vi "Screw Launcher.vi"(9 "Sub Panel":refnum<vi>, 10 "Screw ID":string="Secondary", 11 "Feeder Actor In":refnum<class "Feeder.lvclass">) -> (2 "Nested Actor's Enqueuer":refnum<class "Message Enqueuer.lvclass">, 3 "Feeder Actor Out":refnum<class "Feeder.lvclass">)   [LabVIEW 2018, in "Feeder Actor.lvlib" / "Screw.lvclass"]
uses:
  Screw.lvclass
  <vilib>/ActorFramework/Message Enqueuer/Message Enqueuer.lvclass
  Feeder/Feeder.lvclass
  C:/Program Files/National Instruments/LabVIEW 2018/vi.lib/MGI/Panel Manager/Panel Actor/Panel Actor/Panel Actor.lvclass
  Screw.lvclass/Screw.ctl
  <vilib>/MGI/Panel Manager/Panel/Panel/Subpanel/Subpanel.lvclass
  C:/Program Files/National Instruments/LabVIEW 2018/vi.lib/MGI/Panel Manager/Panel/Panel/Panel.lvclass
  <vilib>/DAQmx/create/channels.llb/DAQmx Create Channel (CO-Pulse Generation-Frequency).vi
  <vilib>/MGI/Panel Manager/Panel/Panel/Subpanel/Subpanel.vi
  <vilib>/DAQmx/configure/timing.llb/DAQmx Timing (Implicit).vi
  <vilib>/MGI/Panel Manager/Panel/Panel.lvlib
  <vilib>/MGI/Panel Manager/Panel Actor/Panel Actor/Panel Actor.lvclass
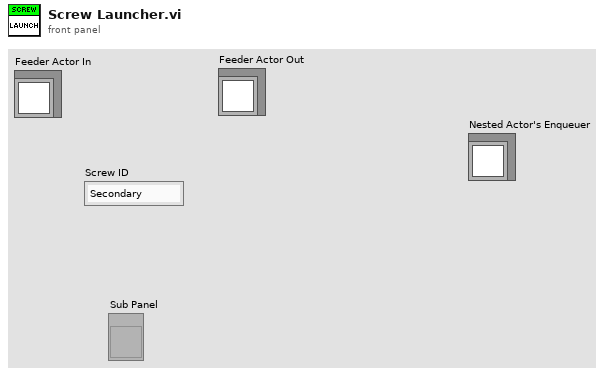
[diagram p1: front panel]
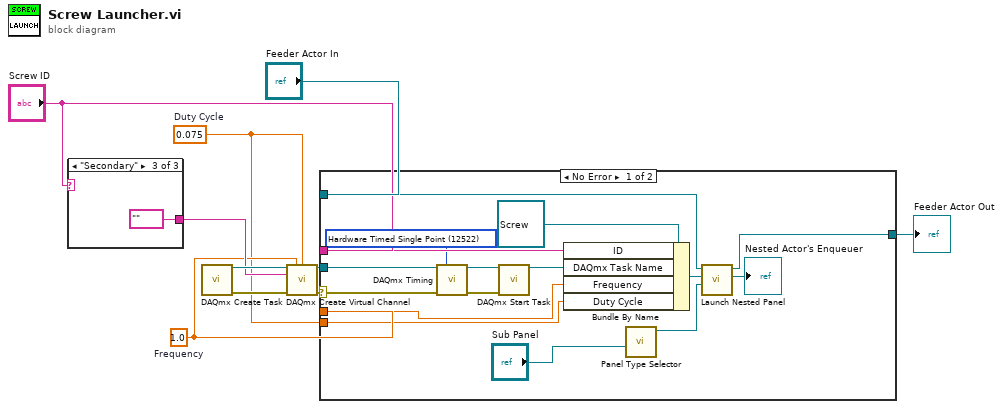
[diagram p0: block diagram]
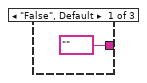
[diagram p2: hidden frame]
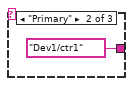
[diagram p3: hidden frame]
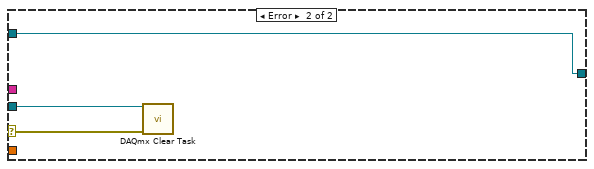
[diagram p4: hidden frame]
diagram:
  w1 = 0.075  # Duty Cycle
  w2 = 1.0  # Frequency
  n1 = case shown="\"Secondary\"" "Screw ID" {
    tunnel: [tag "" ("Counter(s) 2") tag "Dev1/ctr1" ("Counter(s) 2") tag "" ("Counter(s) 2")] -> w5
    frame "False", Default {
    }
    frame "Primary" {
    }
    frame "Secondary" {
    }
  }
  n2 = call <vilib>:"DAQmx Create Task.vi"() -> ("task out"=w7:refnum<k21>, "error out"=w6:errorcluster)  [unwired: 14 in]
  n3 = call-poly <vilib>:"DAQmx Create Virtual Channel.vi"("task in"=w7, "frequency"=w2, "duty cycle"=w1, "counter"=w5, "error in"=w6) -> ("task out"=w3:refnum<k21>, "error out"=w4:errorcluster)  [unwired: 9 in]
  n4 = case shown="No Error" w4 {
    selector: w4 -> [w19 w30]
    tunnel: "Screw ID" -> [w25 _]
    tunnel: "Feeder Actor In" -> [w23 w32]
    tunnel: [w22 w32] -> w9
    tunnel: w3 -> [w18 w31]
    tunnel: w2 -> [w16 _]
    tunnel: w1 -> [w15 _]
    frame No Error {
      w14 = 12522 items=["Finite Samples"=10178, "Continuous Samples"=10123, "Hardware Timed Single Point"=12522] ("sample mode")
      n5 = call-poly <vilib>:"DAQmx Timing.vi"("task/channels in"=w18, "sample mode"=w14, "error in"=w19) -> ("task out"=w21:refnum<k21>, "error out"=w20:errorcluster)  [unwired: 11 in]
      n6 = call <vilib>:"DAQmx Start Task.vi"("task/channels in"=w21, "error in"=w20) -> ("task out"=w17:refnum<k21>)  [unwired: 12 in, 1 out]
      n7 = Bundle By Name(cluster=refnum<class "Screw.lvclass"> refnum ("Feeder Actor.lvlib:Screw.lvclass"), "ID"=w25, "DAQmx Task Name"=w17, "Frequency"=w16, "Duty Cycle"=w15) -> (w26:refnum<class "Screw.lvclass">)
      n8 = call-poly <vilib>:"Panel Type Selector.vi"("Sub Panel"="Sub Panel") -> ("Subpanel Out"=w27:refnum<class "Subpanel.lvclass">)  [unwired: 9 in, 1 out]
      n9 = call <vilib>:"Launch Nested Panel.vi"("Panel"=w27, "Nested Panel Actor"=w26, "Panel Actor in"=w23) -> ("Nested Actor's Enqueuer"=→"Nested Actor's Enqueuer":refnum<class "Message Enqueuer.lvclass">, "Panel Actor out"=w22:refnum<class "Feeder.lvclass">)  [unwired: 5 in, 2 out]
    }
    frame Error {
      n10 = call <vilib>:"DAQmx Clear Task.vi"("task in"=w31, "error in"=w30) -> ()  [unwired: 13 in, 1 out]
    }
  }
  "Feeder Actor Out" <- w9
